vi "epoll_ctl.vi"(6 "epoll data":u64, 7 "epoll events (default: none)":T2[](array[typedef]) items=["EPOLLIN"=1, "EPOLLPRI"=2, "EPOLLOUT"=4, "EPOLLERR"=8, "EPOLLHUP"=16, "EPOLLRDNORM"=64, "EPOLLRDBAND"=128, "EPOLLWRNORM"=256, "EPOLLWRBAND"=512, "EPOLLMSG"=1024, "EPOLLRDHUP"=8192, "EPOLLWAKEUP"=536870912, "EPOLLONESHOT"=1073741824, "EPOLLET"=2147483648], 8 "error in (no error)":errorcluster, 9 "target fd":i32, 10 "operation":T3=1 items=["Add"=1, "Delete"=2, "Modify"=3], 11 "epfd in":i32) -> (0 "error out":errorcluster, 3 "epfd out":i32)   [LabVIEW 2016, in "Linux RT IPC.C.lvlib"]
uses:
  Linux RT IPC.C.lvlib
  Controls/epoll operations.ctl
  Controls/epoll events.ctl
  Controls/epoll event struct.ctl
  Controls/functions.ctl
  <vilib>/NI/NI Linux RT Errno/Linux Errno.lvlib
panel:
  out "event":T1
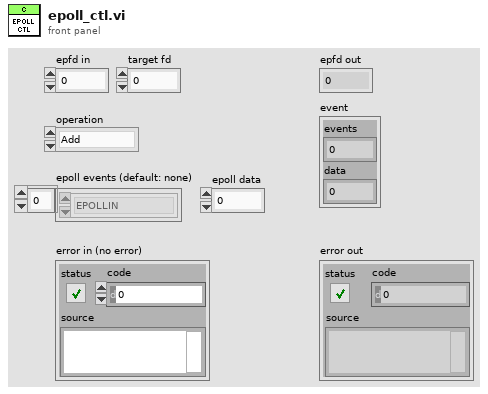
[diagram p1: front panel]
types:
  T1 = typedef "Linux RT IPC.C.lvlib/epoll event struct.ctl" = cluster{"events":u32, "data":u64}
  T2 = typedef "Linux RT IPC.C.lvlib/epoll events.ctl" = u32
  T3 = typedef "Linux RT IPC.C.lvlib/epoll operations.ctl" = u32
  T4 = typedef "Linux RT IPC.C.lvlib/functions.ctl" = enum16{"unspecified", "close", "epoll_create", "epoll_ctl", "epoll_wait", "fstat", "ftruncate", "mkfifo", "mmap", "munmap", "open", "read", "shm_open", "shm_unlink", "timerfd_create", "timerfd_settime", "timerfd_gettime", "write", "unlink"}
  T5 = typedef "Linux Errno.lvlib/errno.ctl" = enum16{"NO ERROR", "EPERM", "ENOENT", "ESRCH", "EINTR", "EIO", "ENXIO", "E2BIG", "ENOEXEC", "EBADF", "ECHILD", "EAGAIN", "ENOMEM", "EACCES", "EFAULT", "ENOTBLK", "EBUSY", "EEXIST", "EXDEV", "ENODEV", "ENOTDIR", "EISDIR", "EINVAL", "ENFILE", "EMFILE", "ENOTTY", "ETXTBSY", "EFBIG", "ENOSPC", "ESPIPE", "EROFS", "EMLINK", "EPIPE", "EDOM", "ERANGE", "EDADLK", "ENAMETOOLONG", "ENOLCK", "ENOSYS", "ENOTEMPTY", "ELOOP", "EWOULDBLOCK", "ENOMSG", "EIDRM", "ECHRNG", "EL2NSYNC", "EL3HLT", "EL3RST", "ELNRNG", "EUNATCH", "ENOCSI", "EL2HLT", "EBADE", "EBADR", "EXFULL", "ENOANO", "EBADRQC", "EBADSLT", "EDEADLOCK", "EBFONT", "ENOSTR", "ENODATA", "ETIME", "ENOSR", "ENONET", "ENOPKG", "EREMOTE", "ENOLINK", "EADV", "ESRMNT", "ECOMM", "EPROTO", "EMULTIHOP", "EDOTDOT", "EBADMSG", "EOVERFLOW", "ENOTUNIQ", "EBADFD", "EREMCHG", "ELIBACC", "ELIBBAD", "ELIBSCN", "ELIBMAX", "ELIBEXEC", "ELISEQ", "ERESTART", "ESTRPIPE", "EUSERS", "ENOTSOCK", "EDESTADDRREQ", "EMSGSIZE", "EPROTOTYPE", "ENOPROTOOPT", "EPROTONOSUPPORT", "ESOCKTNOSUPPORT", "EOPNOTSUPP", "EPFNOSUPPORT", "EAFNOSUPPORT", "EADDRINUSE", "EADDRNOTAVAIL", "ENETDOWN", "ENETUNREACH", "ENETRESET", "ECONNABORTED", "ECONNRESET", "ENOBUFS", "EISCONN", "ENOTCONN", "ESHUTDOWN", "ETOOMANYREFS", "ETIMEDOUT", "ECONNREFUSED", "EHOSTDOWN", "EHOSTUNREACH", "EALREADY", "EINPROGRESS", "ESTALE", "EUCLEAN", "ENOTNAM", "ENAVAIL", "EISNAM", "EREMOTEIO", "EDQUOT", "ENOMEDIUM", "EMEDIUMTYPE", "ECANCELED", "ENOKEY", "EKEYEXPIRED", "EKEYREVOKED", "EKEYREJECTED", "EOWNERDEAD", "ENOTRECOVERABLE", "ERFKILL", "EHWPOISON", "UNDEFINED"}
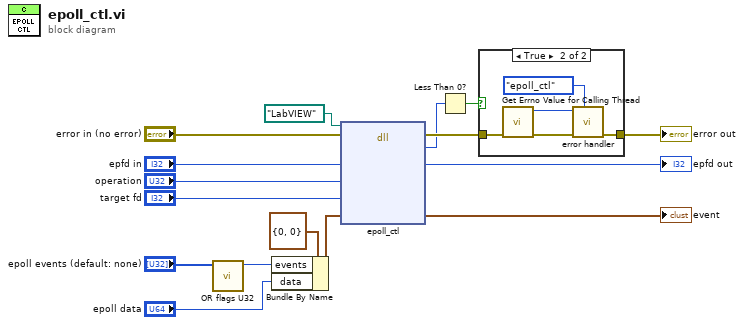
[diagram p0: block diagram]
diagram:
  n1 = call "OR flags U32.vi"("flags"="epoll events (default: none)") -> ("OR'ed flags"=w5:u32)  [unwired: 10 in]
  n2 = Bundle By Name(cluster=T1 {"events"=0, "data"=0} ("event"), "events"=w5, "data"="epoll data") -> (w4:T1)
  n3 = dll-call lib="LabVIEW" fn="epoll_ctl"(path in=path "LabVIEW", error in="error in (no error)", "epfd"="epfd in", "operation"="operation", "fd"="target fd", "event"=w4) -> (error out=w15:errorcluster, "return"=w11:i32, "epfd"=→"epfd out":i32, "event"=→"event":T1)  [unwired: 3 in, 1 out]
  n4 = Less Than 0?(x=w11) -> (x < 0?=w13:bool)
  n5 = case shown="True" w13 {
    tunnel: w15 -> [w17 w22]
    tunnel: [w17 w21] -> w14
    frame False {
    }
    frame True {
      n6 = call <vilib>:"Get Errno Value for Calling Thread.vi"("error in (no error)"=w22) -> ("error out"=w19:errorcluster, "errno"=w20:T5)  [unwired: 9 in]
      n7 = call "error handler.vi"("function (unspecified)"=functions."epoll_ctl" ("function"), "error in (no error)"=w19, "errno"=w20) -> ("error out"=w21:errorcluster)  [unwired: 8 in]
    }
  }
  "error out" <- w14
